vi "Features.vi"(2 "Array in":dbl[](array[numeric]), 3 "Sampling":i32=1) -> (0 "Power Spectrum Graph":cluster{"f0":dbl, "df":dbl, "magnitude":dbl[]}(graph), 1 "Waveform Graph":cluster{i32, dbl, dbl[]}(graph), 5 "Frequency Resolution":dbl, 6 "Sampling Frequency":dbl, 7 "FFT":dbl[](array[numeric]), 9 "abs(FFT)":dbl[](array[numeric]))   [LabVIEW 2023]
uses:
  <vilib>/Analysis/2dsp.llb/Complex FFT.vi
  <vilib>/Waveform/WDTOps.llb/WDT Waveform Duration DBL.vi
  <vilib>/express/express analysis/Spectral/Block/exnSpectralBlock spectral measurements power poly.vi
  <vilib>/express/express analysis/Spectral/Block/exnSpectralBlock spectral measurements power WFM.vi
  <vilib>/express/express analysis/Spectral/XNode/ExpressSpectralMeasurementsBlockNode.xnode
  <vilib>/Analysis/NI_AALPro.lvlib
panel:
  in  "Tab Control":T1(tab)
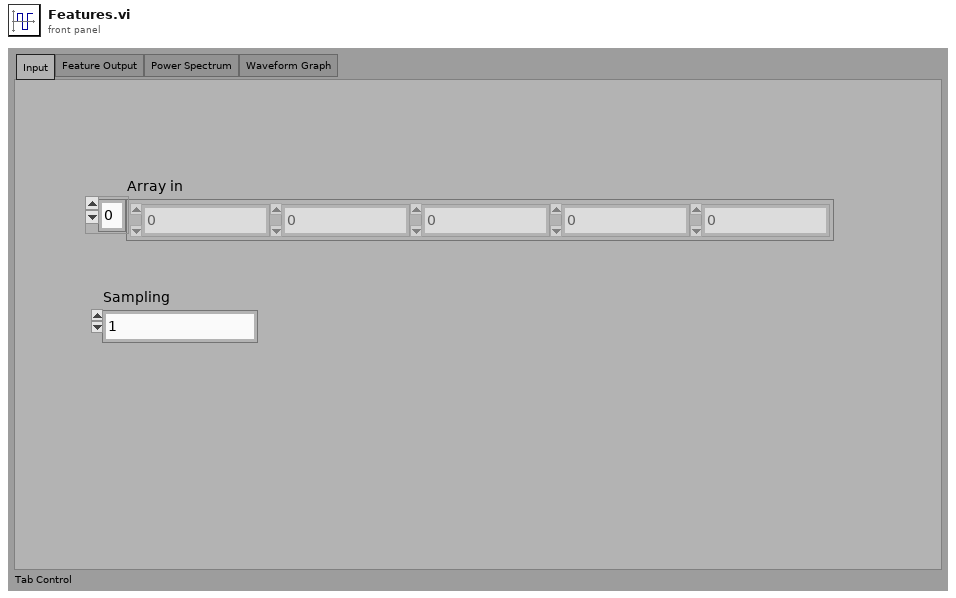
[diagram p1: front panel]
types:
  T1 = enum32{"Input", "Feature Output", "Power Spectrum", "Waveform Graph"}
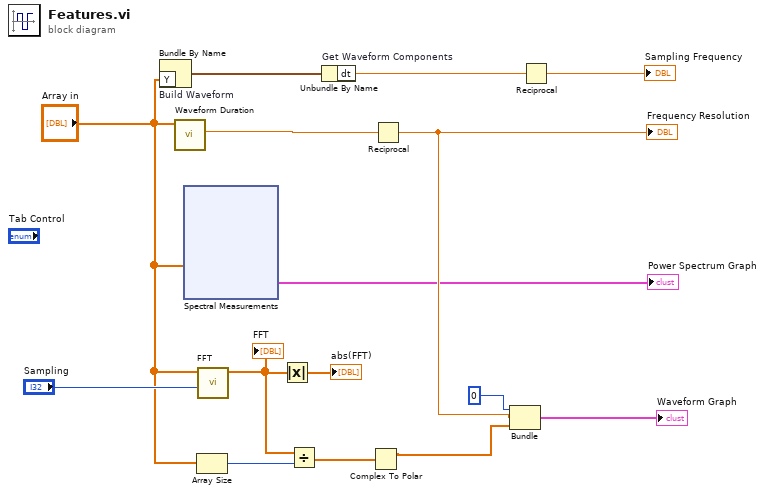
[diagram p0: block diagram]
diagram:
  n1 = Bundle By Name "Build Waveform"("Y"="Array in") -> (w15:waveform(dbl))  [unwired: 1 in]
  n2 = call-poly <vilib>:"Waveform Duration.vi"("waveform in"="Array in") -> ("duration"=w14:dbl)  [unwired: 8 in, 2 out]
  n3 = xnode "Spectral Measurements"("Signals"="Array in") -> ("Power Spectrum"=→"Power Spectrum Graph":cluster{"f0":dbl, "df":dbl, "magnitude":dbl[]})  [unwired: 1 in, 1 out]
  n4 = Array Size(array="Array in") -> (size(s)=w7:i32)
  n5 = call-poly <vilib>:"FFT.vi"("FFT size"="Sampling", "X"="Array in") -> ("FFT {X}"=w8:cdb[])  [unwired: 8 in, 1 out]
  "FFT" <- w8
  n6 = Absolute Value(x=w8) -> (abs(x)=→"abs(FFT)":dbl[])
  n7 = Divide(x=w8, y=w7) -> (x/y=w6:cdb[])
  n8 = Unbundle By Name "Get Waveform Components"(w15) -> ("dt"=w12:dbl)
  n9 = Complex To Polar(r * e^(i*theta)=w6) -> (r=w5:dbl[])  [unwired: 1 out]
  n10 = Reciprocal(x=w14) -> (1/x=w4:dbl)
  "Frequency Resolution" <- w4
  n11 = Bundle "Bundle"(0, w4, w5) -> (→"Waveform Graph":cluster{i32, dbl, dbl[]})  [unwired: 1 in]
  n12 = Reciprocal(x=w12) -> (1/x=→"Sampling Frequency":dbl)
